vi "TelemGUI_v1_4.vi"(0 "Port number":refnum<visa-resource-name>="COM1", 1 "baud rate":u32=38400, 2 "data bits":u16=8 min=5 max=8 step=1, 3 "parity":u16(ring) items=["None", "Odd", "Even", "Mark", "Space"], 4 "stop bits":u16(ring)=10 items=["1.0"=10, "1.5"=15, "2.0"=20], 7 "flow control":u16(ring) items=["None"=0, "XON/XOFF"=1, "RTS/CTS"=2, "DTR/DSR"=4]) -> ()   [LabVIEW 2009]
doc: "McMaster Solar Car Project telemetry graphical front end for Spitfire (2014). Developed for telemetry circuit running firmware revision 6.\n\nINSTRUCTIONS:\n1. In the 'Configuration' tab, select the COM port which the radio is connected to (i.e. - the COM port which enumerated when the UART/receiver module was connected to the PC). If you connected the receiver after opening the GUI, select 'Refresh' from the drop down menu to refresh the COM port list.\n\n2. Set port options. For the current version of the Telemetry hardware using the XCite RF modules use 38400 baud, 8 data bits, parity none, 1 stop bit, flow control none\n\n3. Click on the folder icon next to the log file path dialog box. Select a save location and name for the log file. If you would like to add comments to the log file header, enter these in the 'Notes' dialog box. \n\n4. Select which battery pack is installed in the solar car in the \"Configuration\" tab by clicking the correct radio button (\"Race pack\" or \"Practice pack\"). This selection applies the correct conversion/calibration factors for the current sensor measurement on the battery pack. \n\n5. Click the 'Connect' button. If communication with the telemetry broadcast is successful, the \"heartbeat\" indicator in the window should flash once per full data receipt cycle (approximately once per second). As new data is received from the solar car, the indicators in the various tabs of the front panel will update.\n\n6. To disconnect from the radio link save the data log to file, press the 'Disconnect' button located below the GUI window.\n\n7. If the incorrect COM port was selected, you must first 'Disconnect' before changing the port settings. This also applies if you would like to change the name of the log file. Note that a delay of up to 2 seconds may occur when the 'Disconnect' button is pressed. Once disconnected, change the COM port options and/or the log file path and comment before clicking 'Connect' again.\n\n8. To end execution of the program, first click 'Disconnect' and then click 'Cancel.'\n\nUSAGE NOTES:\n- If the solar car is out of radio range, the telemetry front end displays the most recently received data. The front end will continue to update once the solar car transmitter re-enters radio range.\n\n- In the 'Overview' panel, the displayed 'Battery Charge' is either the charge or discharge capacity, depending on if the battery is charging or discharging. The charge capacity is the estimated state-of-charge of the most charged module in the battery pack; the discharge capacity is the state-of-charge of the least charged module in the battery pack. Both of these values are visible in the 'Battery Details' tab. \n\n- In practice, these two charge values will be different due to battery pack misbalance. A large difference between these two values is undesirable since the battery pack can only be discharged until the discharge capacity reaches 0 and can only be charged until the charge capacity reaches 1.\n\n- Also note that the battery charge is merely an estimate based on a simple battery model. The model predictions are poor above 95% and below 5% state of charge\n\n- The value for \"Range (km)\" is an estimate of the distance that can be travelled at the current rate of power draw from the battery pack before a battery protection system (BPS) trip will occur. The accuracy of this data is untested. This calculation uses the discharge capacity if the battery pack is being discharged, and vice-versa.\n\n- Negative values for range are reported if the battery pack is being charged while the car is driving (i.e. - during regen braking or if the solar array is producing more power than required by the motor).\n\n- Currently \"Economy (Wh/km)\" and \"Range (km)\" are calculated from instantaneous values based on most recently received data. Corrupted radio data will yield nonsensical results (i.e. - at the moment the solar car is leaving or re-entering radio range)."
uses:
  <vilib>/Instr/_visa.llb/VISA Configure Serial Port (Instr).vi
  <vilib>/express/express arith-compare/Formula/XNode/ExpressFormulaBlockNode.xnode
  <vilib>/express/express shared/transition.llb/Waveform Array To Dynamic.vi
  <vilib>/express/express shared/transition.llb/Dynamic To Waveform Array.vi
  <vilib>/express/express shared/ex_Modify Signal Name.vi
  <vilib>/express/express arith-compare/Formula/Block/exnFormulaBlock how many pts in the wave.vi
panel:
  out "Radio heartbeat":bool
  in  "?":T1(tab)
  out "Status message:":string="LabVIEW application is not running! Press Ctrl+R!"
  in  "Cancel Button":bool
  in  "CONNECT":bool
  in  "Battery pack calibration":enum32{"ALPHA", "ZAPPA"}(radio)
  in  "Full path to log file":path
  in  "Notes (appended to log file)":string
  in  "Disconnect":bool
  out "Cruising speed":dbl(slide) scale=0.0..120.0 scale format="%#.0f"
  out "Reverse":bool
  out "MPPT\nTemperature":dbl(slide) scale=0.0..60.0
  out "Net Power Usage (W)":dbl(slide) scale=-1000.0..1000.0
  out "Throttle position":dbl(slide) scale=0.0..1.0 scale format="%#.1f"
  out "Range (km)":dbl format="%.1f"
  out "Battery Charge":dbl(slide) scale=0.0..1.0
  out "Controller \nTemperature":dbl(slide) scale=0.0..60.0
  out "Battery\nTemperature":dbl(slide) scale=0.0..60.0
  out "Aux Error":bool
  out "Aux Low":bool
  out "Aux OK":bool
  out "Pack Hi":bool
  out "Pack Low":bool
  out "Pack OK":bool
  out "Array Amps":dbl format="%.1f"
  out "Motor Amps":dbl format="%.1g"
  out "Motor Power (W)":dbl(slide) scale=0.0..2000.0
  out "Array Power (W)":dbl(slide) scale=0.0..1200.0
  out "Bus Voltage (V)":dbl format="%.1f"
  out "Economy (Wh/km)":dbl format="%.1f"
  out "Speed (km/h)":dbl(knob) scale=0.0..100.0
  out "High temp":bool
  out "Over voltage":bool
  out "Under voltage":bool
  out "Min ID":i8 format="%02x"
  out "Max ID":i8 format="%02x"
  out "Min voltage":dbl format="%.2f"
  out "Max voltage":dbl format="%.2f"
  out "NET battery power (W)":dbl format="%.1f"
  out "MAIN Bus (A)":dbl format="%.1f"
  out "MAIN Bus (V)":dbl format="%.1f"
  out "Error":bool
  out "Low":bool
  out "OK":bool
  out "Max temp (ºC)":dbl(slide) scale=0.0..60.0
  out "AUX Bus (V)":dbl format="%.2f"
  out "Cell Voltages (V)":dbl[](array[numeric]) format="%.2f"
  out "Charge\nCapacity":dbl(slide) scale=0.0..1.0
  out "Discharge\nCapacity":dbl(slide) scale=0.0..1.0
  out "Voltage":dbl[](array[numeric]) format="%.2f"
  out "Temp":dbl[](array[numeric])
  out "BPS total voltage":dbl
  out "MPPT Temp (ºC)":dbl
  out "Power (W)":dbl format="%0.1f"
  out "Current (A)":dbl format="%0.1f"
  out "Voltage (V)":dbl format="%0.1f"
  out "MPPT Temp (ºC)":dbl
  out "Power (W)":dbl format="%0.1f"
  out "Current (A)":dbl format="%0.1f"
  out "Voltage (V)":dbl format="%0.1f"
  out "MPPT Temp (ºC)":dbl
  out "Power (W)":dbl format="%0.1f"
  out "Current (A)":dbl format="%0.1f"
  out "Voltage (V)":dbl format="%0.1f"
  out "MPPT Temp (ºC)":dbl
  out "Power (W)":dbl format="%0.1f"
  out "Current (A)":dbl format="%0.1f"
  out "Voltage (V)":dbl format="%0.1f"
  out "NET OUTPUT (W)":dbl format="%6.1f"
  out "Output current (A)":dbl format="%.1f"
  out "Output voltage (V)":dbl format="%.1f"
  out "Drive Velocity":dbl
  out "Drive Current":dbl format="%.2f"
  out "DSP Temp":dbl
  out "HS Temp":dbl
  out "RPM":dbl
  out "Bus Curr":dbl format="%.1f"
  out "Bus Volt":dbl format="%.1f"
  out "ArrayCurr":dbl
  out "AuxCell":dbl[](array[numeric])
  out "Temp":dbl[](array[numeric])
  out "Volt Out":dbl[](array[numeric])
  out "Curr In":dbl[](array[numeric])
  out "Volt In":dbl[](array[numeric])
  out "Current":dbl
  out "Temp":dbl[](array[numeric])
  out "Radio receive buffer":string
  out "Volt":dbl[](array[numeric])
  out "Selected COM port":refnum<visa-resource-name>
  out "COM error out":errorcluster
  out "Logfile handle":refnum<file>
  # "2014 Telemetry GUI v1.4"
  # "For additional information select File >> VI Properties >> Documentation"
  # "NOTE - Default port settings are:\nBaud rate: 38400\nData bits: 8\nParity: none\nStop bits: 1\nFlow control: none"
  # "Voltage Status"
  # "Pack module readings"
  # "Pack status and warnings"
  # "0x00"
  # "0x01"
  # "0x02"
  # "0x03"
  # "0x04"
  # "0x05"
  # "0x06"
  # "0x07"
  # "0x08"
  # "0x09"
  # "0x0A"
  # "0x0B"
  # "0x0C"
  # "0x0D"
  # "0x0E"
  # "0x0F"
  # "0x10"
  # "0x11"
  # "Cell 0"
  # "0x12"
  # "Cell 1"
  # "0x13"
  # "Cell 2"
  # "0x14"
  # "0x15"
  # "Cell 3"
  # "0x16"
  # "0x17"
  # "0x18"
  # "0x19"
  # "BANK A"
  # "BANK B"
  # "BANK A"
  # "BANK B"
  # "BANK C"
  # "BANK D"
  # "BANK C"
  # "BANK D"
  # "Raw analog data"
  # "MPPT raw data"
  # "BPS raw data"
  # "0001"
  # "0010"
  # "0x00"
  # "0011"
  # "0x01"
  # "0100"
  # "0x02"
  # "0x03"
  # "0x04"
  # "Tritium/Drive raw data"
  # "0x05"
  # "0x06"
  # "0x07"
  # "0x08"
  # "0x09"
  # "0x0A"
  # "0x0B"
  # "0x0C"
  # "0x0D"
  # "0x0E"
  # "0x0F"
  # "0x10"
  # "0x11"
  # "0x12"
  # "0x13"
  # "0x14"
  # "0x15"
  # "0x16"
  # "0x17"
  # "0x18"
  # "0x19"
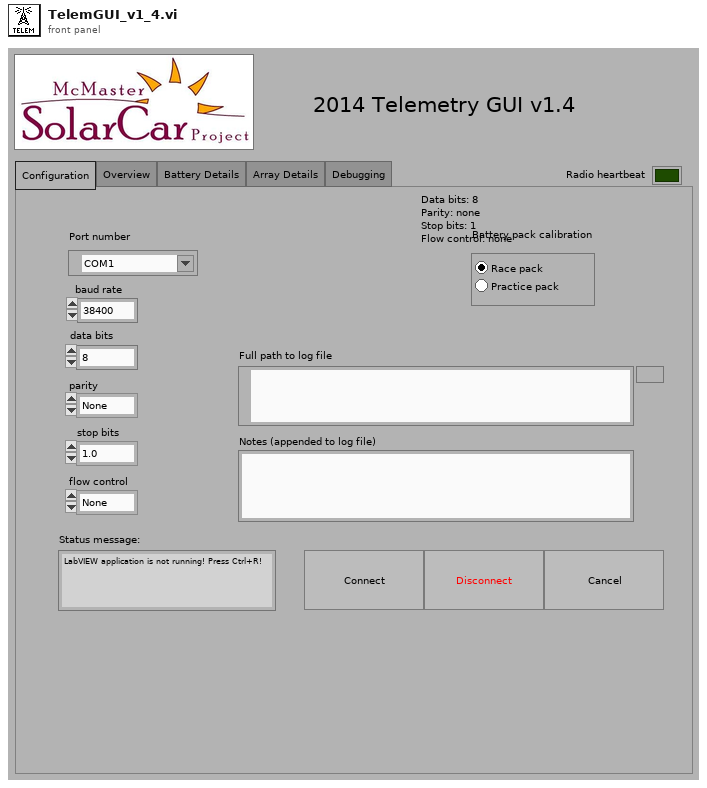
[diagram p1: front panel]
types:
  T1 = enum32{"Configuration", "Overview", "Battery Details", "Array Details", "Debugging"}
  T2 = enum16{"open", "replace", "create", "open or create", "replace or create", "replace or create with confirmation"}
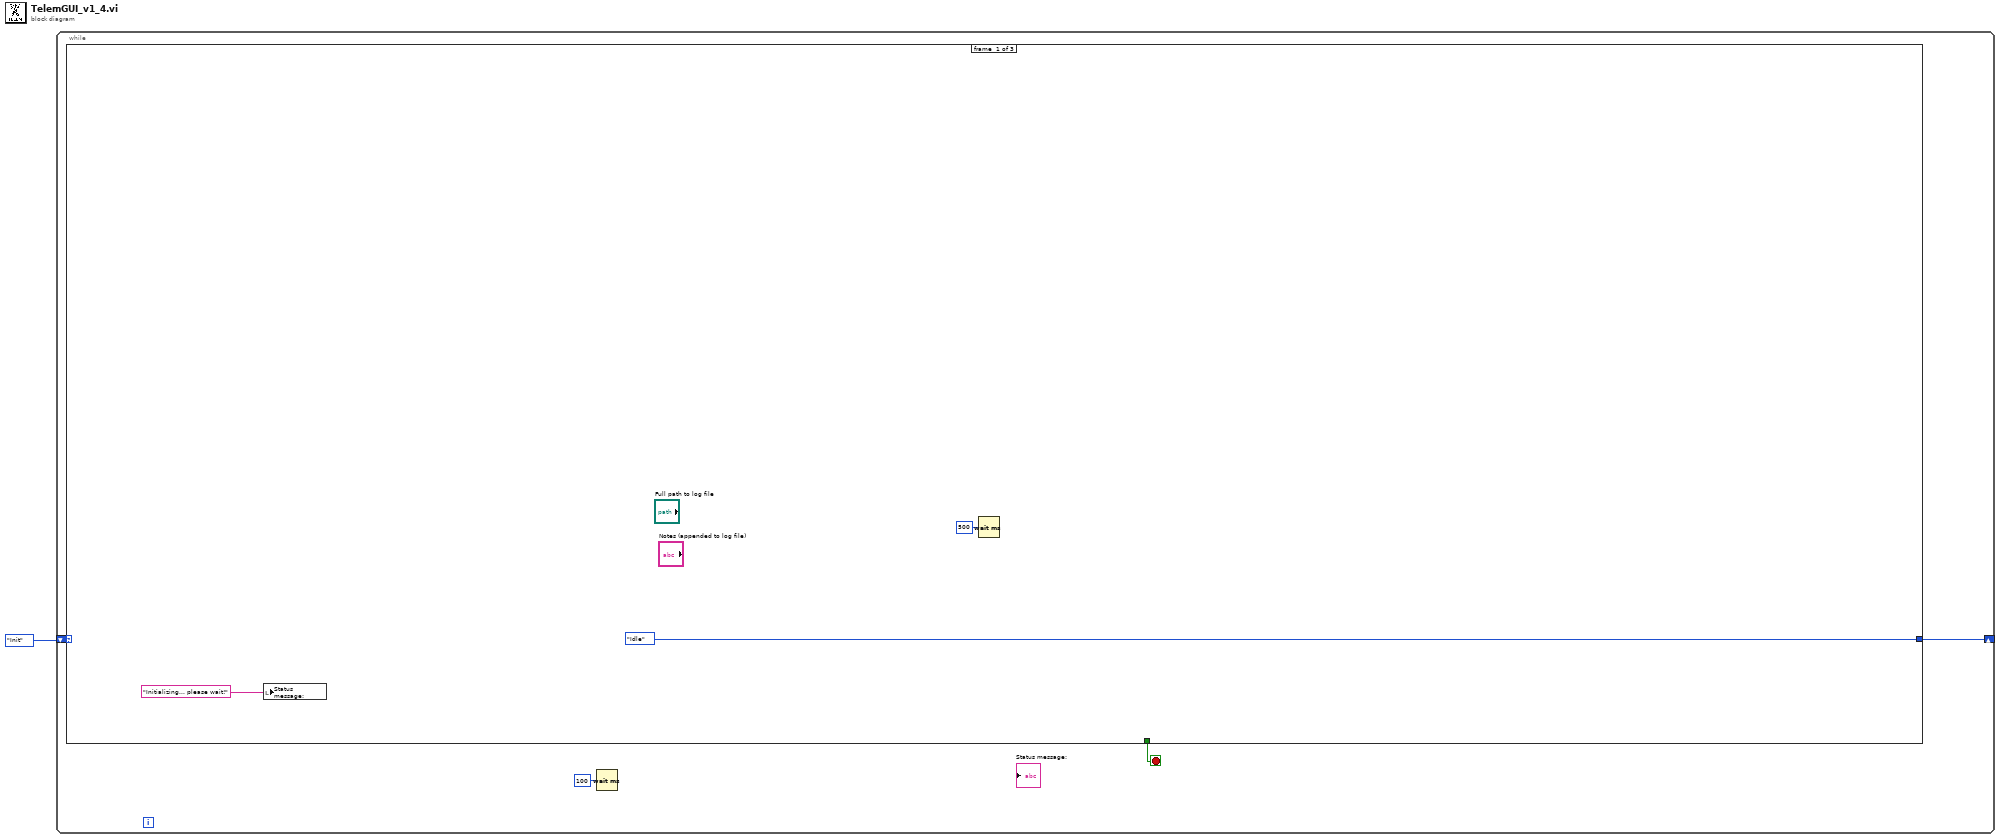
[diagram p0: block diagram]
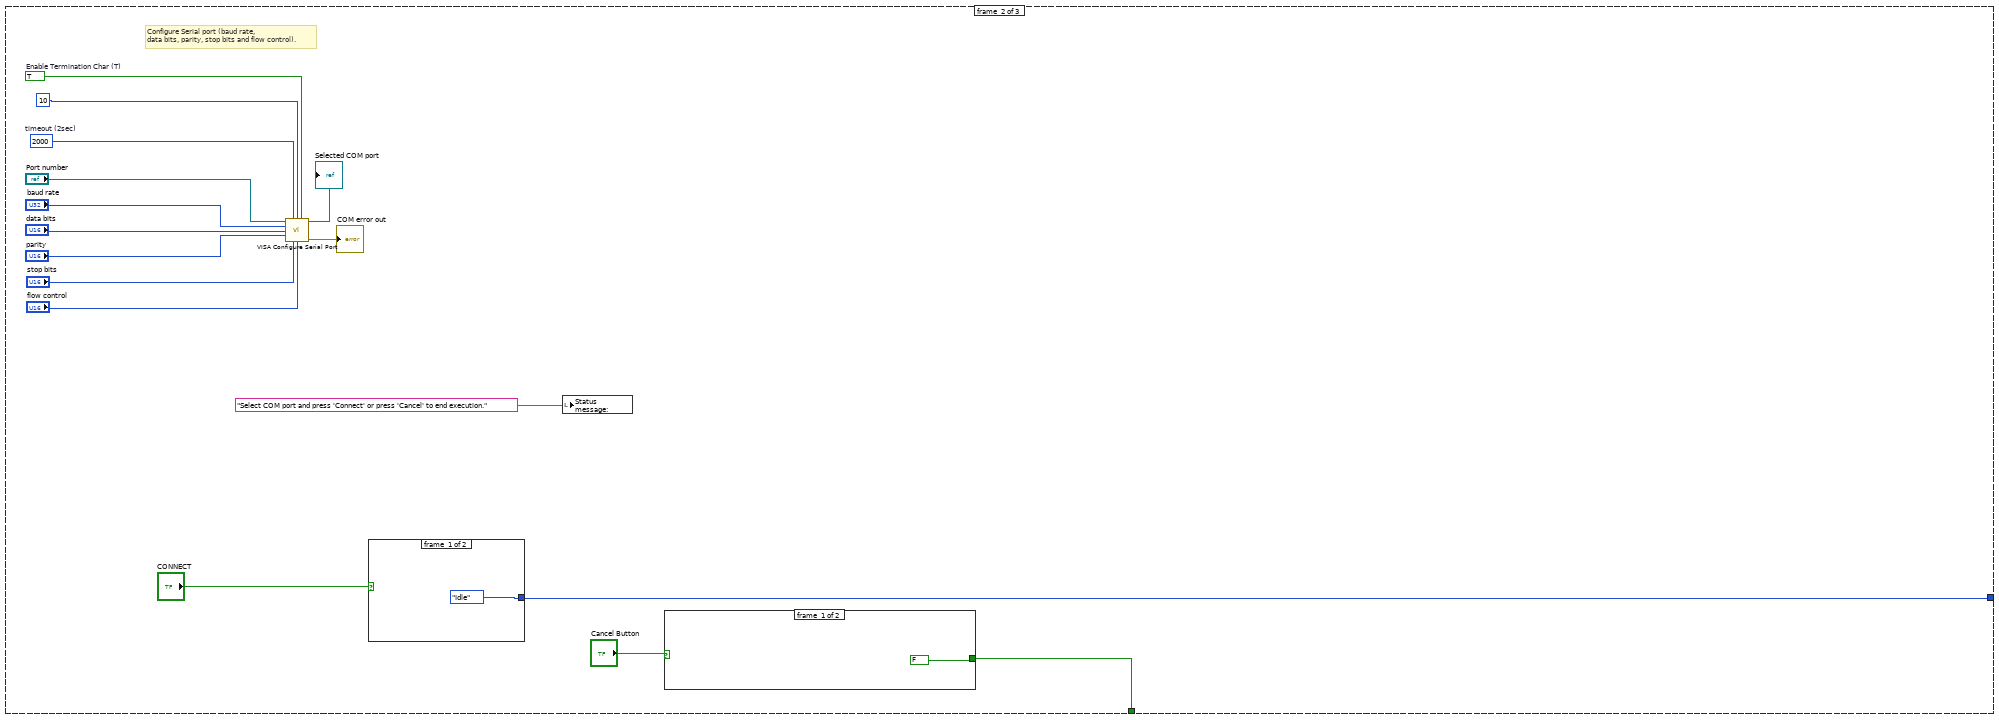
[diagram p2: hidden frame]
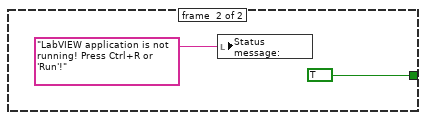
[diagram p3: hidden frame]
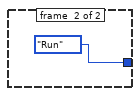
[diagram p4: hidden frame]
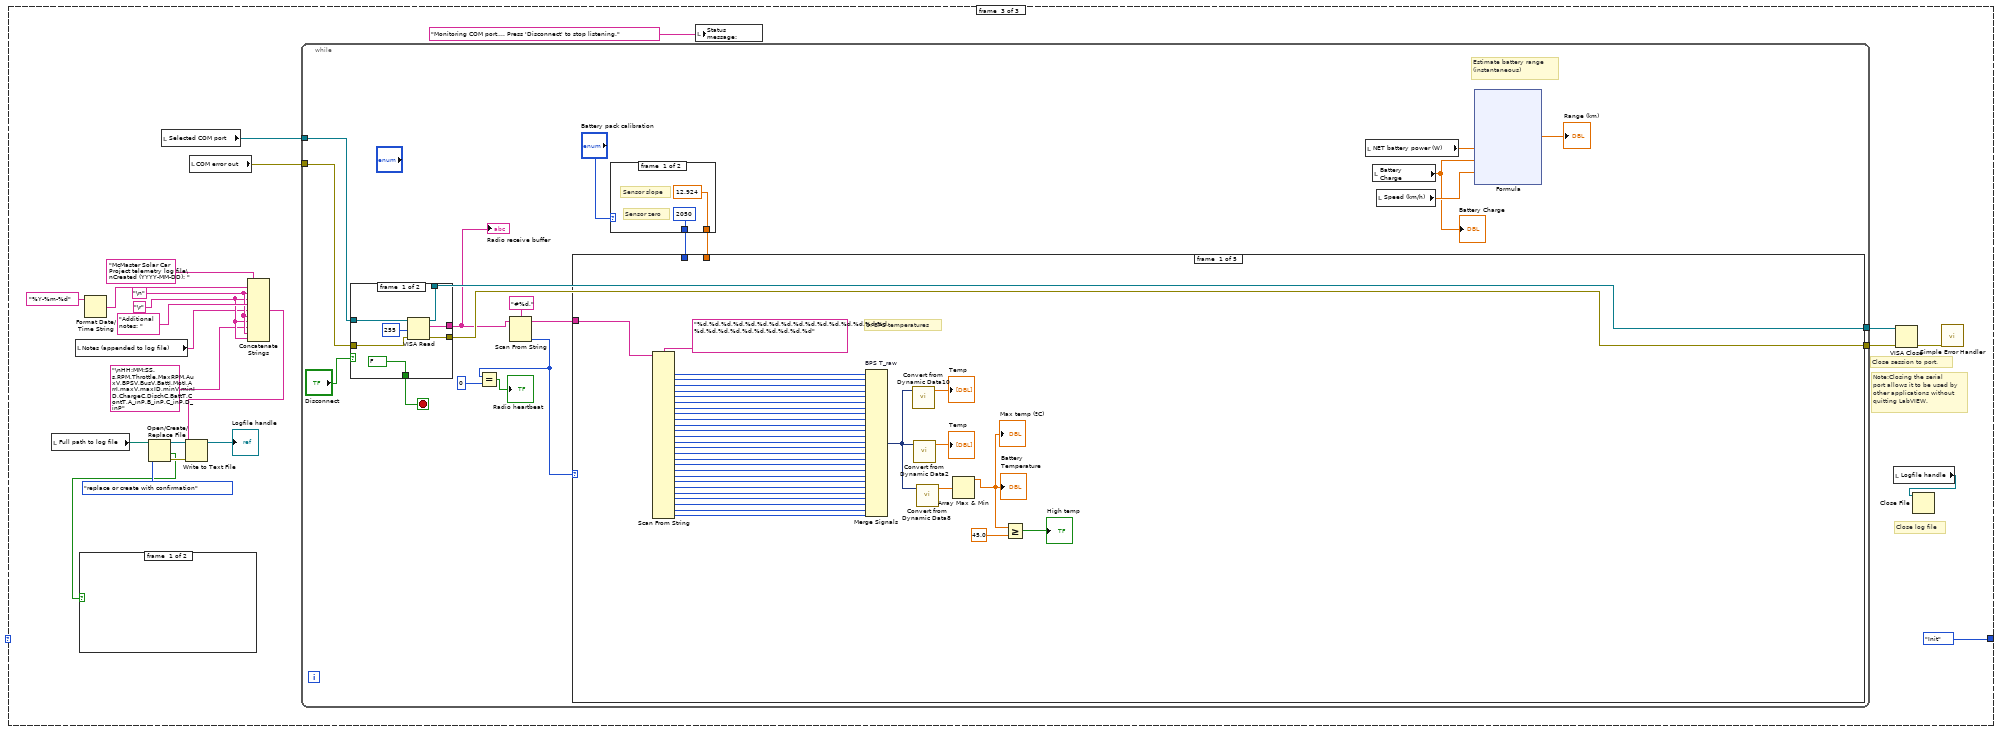
[diagram p5: hidden frame]
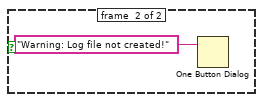
[diagram p6: hidden frame]
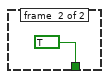
[diagram p7: hidden frame]
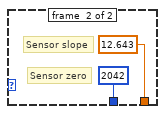
[diagram p8: hidden frame]
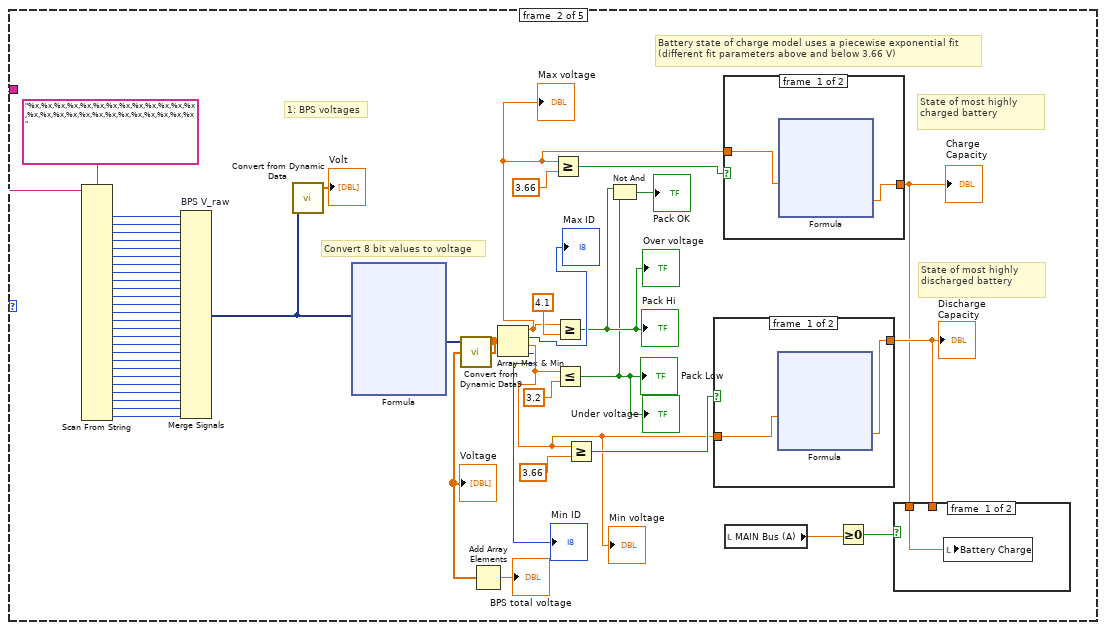
[diagram p9: hidden frame]
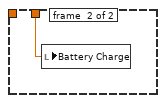
[diagram p10: hidden frame]
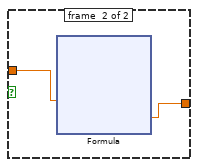
[diagram p11: hidden frame]
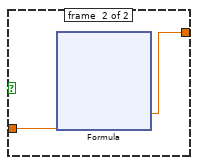
[diagram p12: hidden frame]
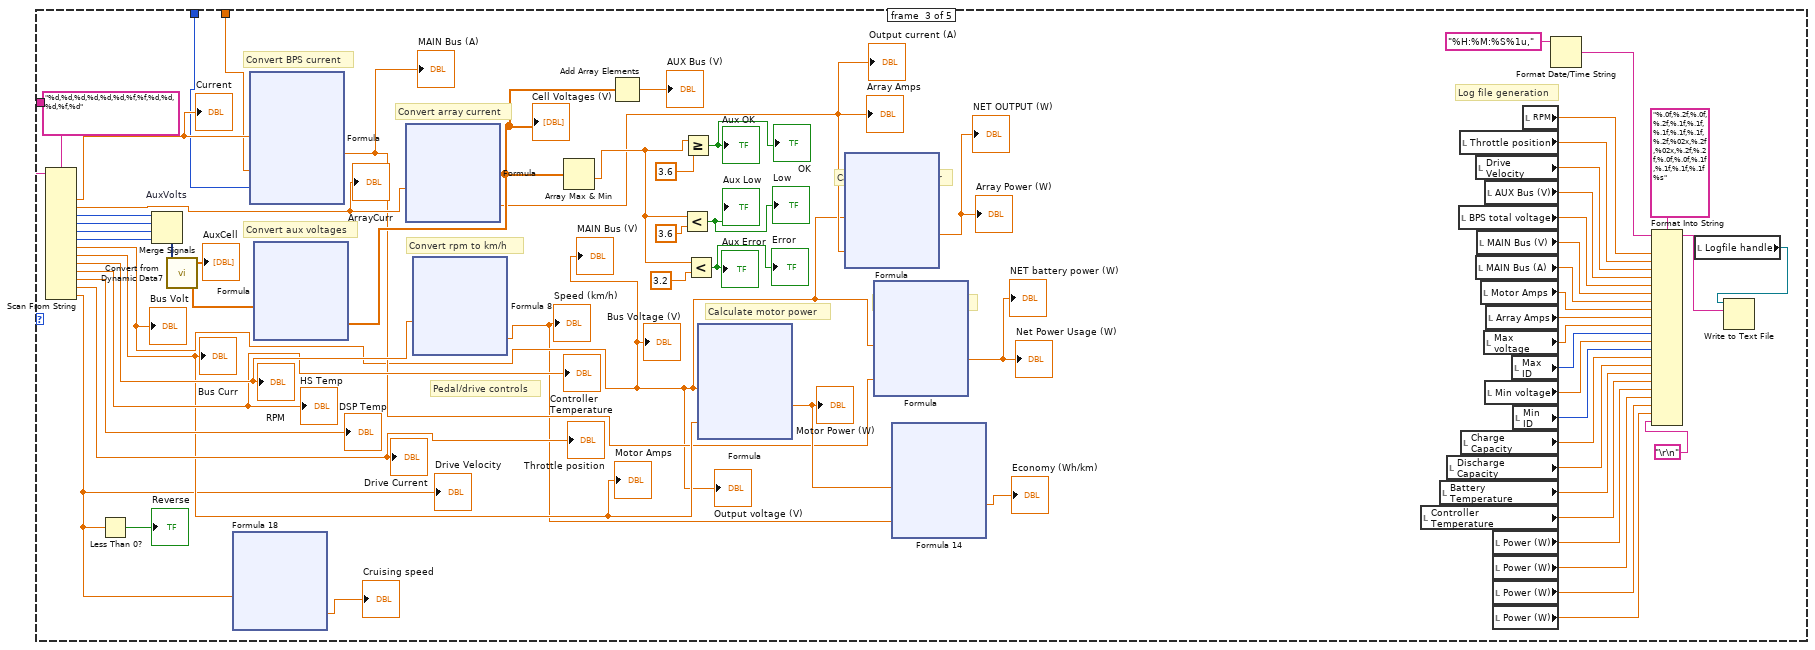
[diagram p13: hidden frame]
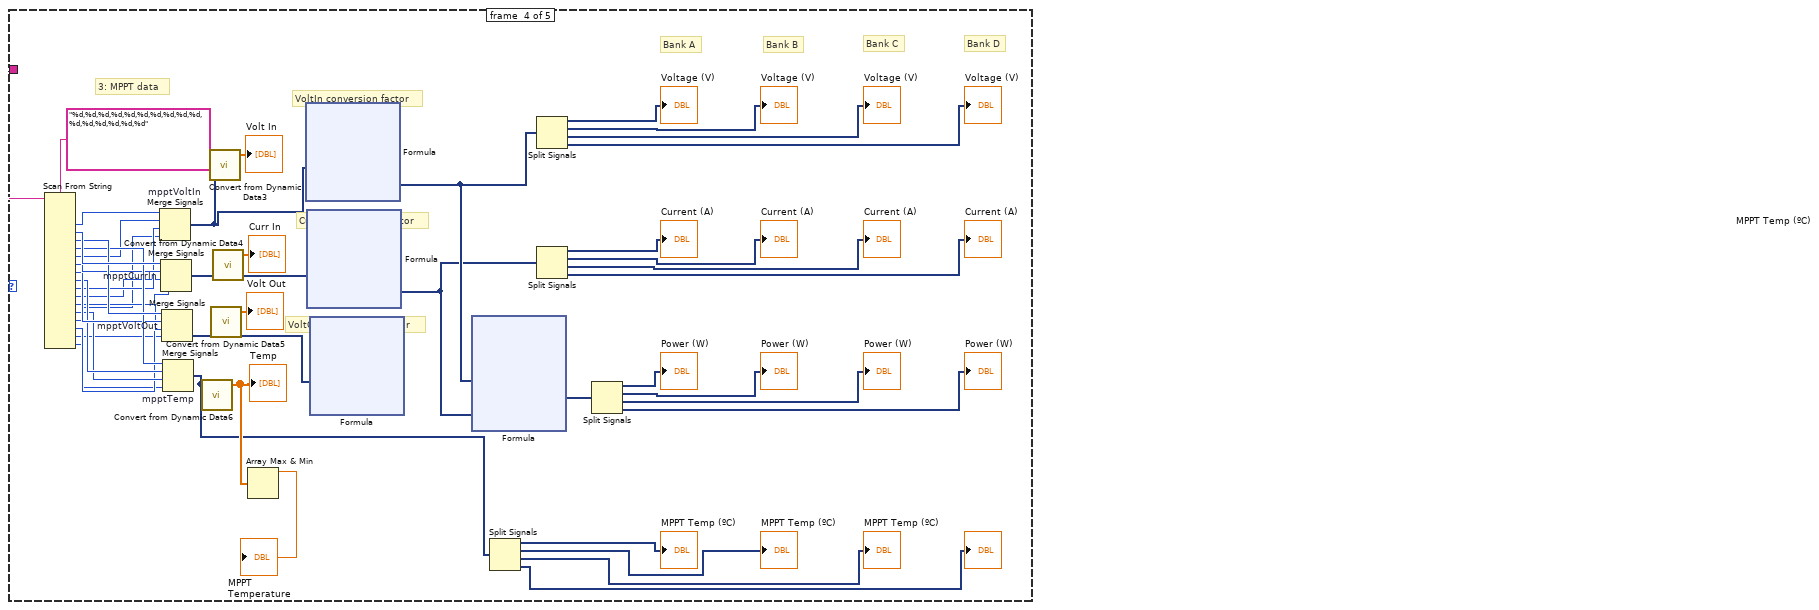
[diagram p14: hidden frame]
diagram:
  n1 = while {
    shift-right: [w4] -> _
    shift-left: enum16{"Init", "Idle", "Run"}."Init" -> [w5]
    stop <- w2 stop-if-true
    n2 = case shown="\"Run\"" w5 {
      tunnel: [enum16{"Init", "Idle", "Run"}."Idle" w23 enum16{"Init", "Idle", "Run"}."Init"] -> w4
      tunnel: [_ w20 _] -> w2
      frame #0 {
        n3 = local write "Status message:"("Initializing... please wait!" ("Status message:")) -> ()
        n4 = Wait (ms)(milliseconds to wait=u32 500) -> ()  [unwired: 1 out]
      }
      frame #1 {
        w15 = TRUE  # Enable Termination Char (T)
        w14 = u32 2000  # timeout (2sec)
        # "Configure Serial port (baud rate,\ndata bits, parity, stop bits and flow control)."
        n5 = call-poly "VISA Configure Serial Port"("VISA resource name"="Port number", "timeout (10sec)"=w14, "termination char\n(0xA = '\\n' = LF)"=10, "Enable Termination\nChar (T)"=w15, "baud rate (9600)"="baud rate", "data bits (8)"="data bits", "parity (0:none)"="parity", "stop bits (10: 1 bit)"="stop bits", "flow control (0:none)"="flow control") -> ("VISA resource name out"=→"Selected COM port":refnum<visa-resource-name>, "error out"=→"COM error out":errorcluster)  [unwired: 5 in]
        n6 = case shown="False" "CONNECT" {
          tunnel: [enum16{"Init", "Idle", "Run"}."Idle" enum16{"Init", "Idle", "Run"}."Run"] -> w23
          frame #0 {
          }
          frame #1 {
          }
        }
        n7 = local write "Status message:"("Select COM port and press 'Connect' or press 'Cancel' to end execution." ("Status")) -> ()
        n8 = case shown="True" "Cancel Button" {
          tunnel: [FALSE TRUE] -> w20
          frame #0 {
          }
          frame #1 {
            n9 = local write "Status message:"("LabVIEW application is not running! Press Ctrl+R or 'Run'!" ("Status")) -> ()
          }
        }
      }
      frame #2 {
        w39 = "\n"
        w38 = "\r"
        # "Close log file"
        # "Note:Closing the serial port allows it to be used by other applications without\nquitting LabVIEW."
        # "Close session to port."
        n10 = local read "Full path to log file"() -> (w45:path)
        n11 = local read "Notes (appended to log file)"() -> (w34:string)
        n12 = Format Date/Time String(time format string (%c)="%Y-%m-%d") -> (date/time string=w41:string)  [unwired: 2 in]
        n13 = Open/Create/Replace File(file path (use dialog)=w45, operation (0:open)=T2."replace or create with confirmation") -> (refnum out=w48:refnum<file>, cancelled=w44:bool, error out=w47:errorcluster)  [unwired: 4 in]
        n14 = case shown="True" w44 {
          frame #0 {
          }
          frame #1 {
            n15 = One Button Dialog ("Log creation cancelled")(message="Warning: Log file not created!") -> ()  [unwired: 1 in, 1 out]
          }
        }
        n16 = local read "Selected COM port"() -> (w37:refnum<visa-resource-name>)
        n17 = local read "COM error out"() -> (w36:errorcluster)
        n18 = Concatenate Strings("McMaster Solar Car Project telemetry log file\nCreated (YYYY-MM-DD): ", w41, w39, w38, "Additional notes: " ("string"), w34, w39, w38, "\nHH:MM:SS.s,RPM,Throttle,MaxRPM,AuxV,BPSV,BusV,BattI,MotI,ArrI,maxV,maxID,minV,minID,ChargeC,DischC,BattT,ContT,A_inP,B_inP,C_inP,D_inP" ("string"), w39, w38) -> (w35:string)
        n19 = Write to Text File(file (use dialog)=w48, text=w35, error in=w47) -> (refnum out=→"Logfile handle":refnum<file>)  [unwired: 1 in, 2 out]
        n20 = while {
          tunnel: [w58] -> w50
          tunnel: [w59] -> w51
          tunnel: w37 -> [w55]
          tunnel: w36 -> [w54]
          stop <- w56 stop-if-true
          # "Estimate battery range\n(instantaneous)"
          n21 = case shown="False" "Disconnect" {
            tunnel: w55 -> [w78 _]
            tunnel: w54 -> [w77 _]
            tunnel: [w76 _] -> w59
            tunnel: [w75 _] -> w58
            tunnel: [w74 _] -> w57
            tunnel: [FALSE TRUE] -> w56
            frame #0 {
              n22 = VISA Read(VISA resource name=w78, byte count=255, error in (no error)=w77) -> (VISA resource name out=w76:refnum<visa-resource-name>, read buffer=w74:string, error out=w75:errorcluster)  [unwired: 1 out]
            }
            frame #1 {
            }
          }
          "Radio receive buffer" <- w57
          n23 = Scan From String(format string="#%d,", input string=w57) -> (remaining string=w71:string, output 1=w70:i32)  [unwired: 3 in, 2 out]
          n24 = Equal?(x=w70, y=0) -> (x = y?=→"Radio heartbeat":bool)
          n25 = case shown="\"ALPHA\", Default" "Battery pack calibration" {
            tunnel: [12.924 12.643] -> w66
            tunnel: [2050 2042] -> w65
            frame #0 {
              # "Sensor zero"
              # "Sensor slope"
            }
            frame #1 {
              # "Sensor zero"
              # "Sensor slope"
            }
          }
          n26 = case shown="2" w70 {
            tunnel: w71 -> [w131 w180 w425 w557 _]
            tunnel: w66 -> [_ _ w400 _ _]
            tunnel: w65 -> [_ _ w399 _ _]
            frame #0 {
              # "0: BPS temperatures"
              n27 = Scan From String(format string="%d,%d,%d,%d,%d,%d,%d,%d,%d,%d,%d,%d,%d,%d,%d,%d,%d,%d,%d,%d,%d,%d,%d,%d,%d,%d", input string=w131) -> (output 1=w129:i32, output 2=w128:i32, output 3=w127:i32, output 4=w126:i32, output 5=w125:i32, output 6=w124:i32, output 7=w123:i32, output 8=w122:i32, output 9=w121:i32, output 10=w120:i32, output 11=w119:i32, output 12=w118:i32, output 13=w117:i32, output 14=w116:i32, output 15=w115:i32, output 16=w114:i32, output 17=w113:i32, output 18=w112:i32, output 19=w111:i32, output 20=w110:i32, output 21=w109:i32, output 22=w108:i32, output 23=w107:i32, output 24=w104:i32, output 25=w106:i32, output 26=w105:i32)  [unwired: 28 in, 3 out]
              n28 = Merge Signals "BPS T_raw"(w129, w128, w127, w126, w125, w124, w123, w122, w121, w120, w119, w118, w117, w116, w115, w114, w113, w112, w111, w110, w109, w108, w107, w104, w106, w105) -> (w102:dynamicdata)
              n29 = call "Convert from Dynamic Data10"("Dynamic Data Type"=w102) -> ("Array"=→"Temp":dbl[])  [unwired: 3 in]
              n30 = call "Convert from Dynamic Data2"("Dynamic Data Type"=w102) -> ("Array"=→"Temp":dbl[])  [unwired: 3 in]
              n31 = call "Convert from Dynamic Data8"("Dynamic Data Type"=w102) -> ("Array"=w97:dbl[])  [unwired: 3 in]
              n32 = Array Max & Min(array=w97) -> (max value=w100:dbl)  [unwired: 3 out]
              "Battery\nTemperature" <- w100
              "Max temp (ºC)" <- w100
              n33 = Greater Or Equal?(x=w100, y=45.0) -> (x >= y?=→"High temp":bool)
            }
            frame #1 {
              # "State of most highly discharged battery"
              # "State of most highly charged battery"
              # "Battery state of charge model uses a piecewise exponential fit\n(different fit parameters above and below 3.66 V)"
              # "1: BPS voltages"
              # "Convert 8 bit values to voltage"
              n34 = Scan From String(format string="%x,%x,%x,%x,%x,%x,%x,%x,%x,%x,%x,%x,%x,%x,%x,%x,%x,%x,%x,%x,%x,%x,%x,%x,%x,%x", input string=w180) -> (output 1=w179:i32, output 2=w178:i32, output 3=w177:i32, output 4=w176:i32, output 5=w175:i32, output 6=w174:i32, output 7=w173:i32, output 8=w172:i32, output 9=w171:i32, output 10=w170:i32, output 11=w169:i32, output 12=w168:i32, output 13=w167:i32, output 14=w166:i32, output 15=w165:i32, output 16=w164:i32, output 17=w163:i32, output 18=w162:i32, output 19=w161:i32, output 20=w160:i32, output 21=w159:i32, output 22=w154:i32, output 23=w158:i32, output 24=w157:i32, output 25=w156:i32, output 26=w155:i32)  [unwired: 28 in, 3 out]
              n35 = Merge Signals "BPS V_raw"(w179, w178, w177, w176, w175, w174, w173, w172, w171, w170, w169, w168, w167, w166, w165, w164, w163, w162, w161, w160, w159, w154, w158, w157, w156, w155) -> (w153:dynamicdata)
              n36 = call "Convert from Dynamic Data"("Dynamic Data Type"=w153) -> ("Array"=→"Volt":dbl[])  [unwired: 3 in]
              n37 = xnode "Formula"("X1"=w153) -> ("Result"=w151:dynamicdata)  [unwired: 1 in, 1 out]
              n38 = call "Convert from Dynamic Data9"("Dynamic Data Type"=w151) -> ("Array"=w133:dbl[])  [unwired: 3 in]
              "Voltage" <- w133
              n39 = Add Array Elements(numeric array=w133) -> (sum=→"BPS total voltage":dbl)
              n40 = Array Max & Min(array=w133) -> (max value=w143:dbl, max index (indices)=→"Max ID":i32, min value=w142:dbl, min index (indices)=→"Min ID":i32)
              "Max voltage" <- w143
              "Min voltage" <- w142
              n41 = Greater Or Equal?(x=w143, y=3.66) -> (x >= y?=w144:bool)
              n42 = Greater Or Equal?(x=w143, y=4.1) -> (x >= y?=w139:bool)
              "Pack Hi" <- w139
              "Over voltage" <- w139
              n43 = Less Or Equal?(x=w142, y=3.2) -> (x <= y?=w138:bool)
              "Pack Low" <- w138
              "Under voltage" <- w138
              n44 = Greater Or Equal?(x=w142, y=3.66) -> (x >= y?=w146:bool)
              n45 = Not And(1:w138, 2:w139) -> (0:→"Pack OK":bool)
              n46 = case shown="False" w146 {
                tunnel: w142 -> [w205 w215]
                tunnel: [w204 w214] -> w135
                frame #0 {
                  n47 = xnode "Formula"("X1"=w205) -> ("Result"=w204:dbl)  [unwired: 1 in, 1 out]
                }
                frame #1 {
                  n48 = xnode "Formula"("X1"=w215) -> ("Result"=w214:dbl)  [unwired: 1 in, 1 out]
                }
              }
              "Discharge\nCapacity" <- w135
              n49 = case shown="False" w144 {
                tunnel: [w185 w195] -> w134
                tunnel: w143 -> [w184 w194]
                frame #0 {
                  n50 = xnode "Formula"("X1"=w184) -> ("Result"=w185:dbl)  [unwired: 1 in, 1 out]
                }
                frame #1 {
                  n51 = xnode "Formula"("X1"=w194) -> ("Result"=w195:dbl)  [unwired: 1 in, 1 out]
                }
              }
              "Charge\nCapacity" <- w134
              n52 = local read "MAIN Bus (A)"() -> (w137:dbl)
              n53 = Greater Or Equal To 0?(x=w137) -> (x >= 0?=w136:bool)
              n54 = case shown="True" w136 {
                tunnel: w135 -> [_ w183]
                tunnel: w134 -> [w182 _]
                frame #0 {
                  n55 = local write "Battery Charge"(w182) -> ()
                }
                frame #1 {
                  n56 = local write "Battery Charge"(w183) -> ()
                }
              }
            }
            frame #2 {
              # "Log file generation"
              # "Calculate array power"
              # "Battery (net) power"
              # "Calculate motor power"
              # "Convert rpm to km/h"
              # "Pedal/drive controls"
              # "Convert aux voltages"
              # "Convert array current"
              # "Convert BPS current"
              n57 = Scan From String(format string="%d,%d,%d,%d,%d,%d,%f,%f,%d,%d,%d,%f,%d", input string=w425) -> (output 1=w420:dbl, output 2=w417:dbl, output 3=w424:i32, output 4=w423:i32, output 5=w422:i32, output 6=w421:i32, output 7=w392:dbl, output 8=w410:dbl, output 9=w415:dbl, output 10=→"HS Temp" →"Controller \nTemperature":dbl, output 11=→"DSP Temp":dbl, output 12=→"Drive Current" →"Throttle position":dbl, output 13=w402:dbl)  [unwired: 15 in, 3 out]
              "Current" <- w420
              "ArrayCurr" <- w417
              "Bus Volt" <- w392
              "Bus Curr" <- w410
              "RPM" <- w415
              "Drive Velocity" <- w402
              "Motor Amps" <- w410
              "Bus Voltage (V)" <- w392
              "Output voltage (V)" <- w392
              "MAIN Bus (V)" <- w392
              n58 = Less Than 0?(x=w402) -> (x < 0?=→"Reverse":bool)
              n59 = Merge Signals "AuxVolts"(w424, w423, w422, w421) -> (w419:dynamicdata)
              n60 = call "Convert from Dynamic Data7"("Dynamic Data Type"=w419) -> ("Array"=w418:dbl[])  [unwired: 3 in]
              "AuxCell" <- w418
              n61 = xnode "Formula 18"("RPM"=w402) -> ("Result"=→"Cruising speed":dbl)  [unwired: 1 in, 1 out]
              n62 = xnode "Formula"("battADC"=w420, "hallSlope"=w400, "hallZero"=w399) -> ("Result"=w393:dbl)  [unwired: 1 in, 1 out]
              "MAIN Bus (A)" <- w393
              n63 = xnode "Formula"("X1"=w418) -> ("Result"=w406:dbl[])  [unwired: 1 in, 1 out]
              "Cell Voltages (V)" <- w406
              n64 = xnode "Formula"("ArrayADC"=w417) -> ("Result"=w397:dbl)  [unwired: 1 in, 1 out]
              "Array Amps" <- w397
              "Output current (A)" <- w397
              n65 = xnode "Formula 8"("RPM"=w415) -> ("Result"=w390:dbl)  [unwired: 1 in, 1 out]
              "Speed (km/h)" <- w390
              n66 = Array Max & Min(array=w406) -> (min value=w404:dbl)  [unwired: 3 out]
              n67 = Add Array Elements(numeric array=w406) -> (sum=→"AUX Bus (V)":dbl)
              n68 = Less?(x=w404, y=3.6) -> (x < y?=→"Aux Low" →"Low":bool)
              n69 = Greater Or Equal?(x=w404, y=3.6) -> (x >= y?=→"Aux OK" →"OK":bool)
              n70 = Less?(x=w404, y=3.2) -> (x < y?=→"Aux Error" →"Error":bool)
              n71 = xnode "Formula"("BusVolt"=w392, "MotCurr"=w410) -> ("Result"=w409:dbl)  [unwired: 1 in, 1 out]
              "Motor Power (W)" <- w409
              n72 = xnode "Formula"("BusVolt"=w392, "ArrayCurr"=w397) -> ("Result"=→"Array Power (W)" →"NET OUTPUT (W)":dbl)  [unwired: 1 in, 1 out]
              n73 = xnode "Formula"("busVolt"=w392, "battCurr"=w393) -> ("Result"=→"Net Power Usage (W)" →"NET battery power (W)":dbl)  [unwired: 1 in, 1 out]
              n74 = xnode "Formula 14"("MotW"=w409, "Speed"=w390) -> ("Result"=→"Economy (Wh/km)":dbl)  [unwired: 1 in, 1 out]
              n75 = local read "Controller \nTemperature"() -> (w368:dbl)
              n76 = local read "Battery\nTemperature"() -> (w369:dbl)
              n77 = local read "Discharge\nCapacity"() -> (w370:dbl)
              n78 = local read "BPS total voltage"() -> (w382:dbl)
              n79 = local read "Throttle position"() -> (w385:dbl)
              n80 = local read "Charge\nCapacity"() -> (w371:dbl)
              n81 = local read "Drive Velocity"() -> (w384:dbl)
              n82 = local read "MAIN Bus (A)"() -> (w380:dbl)
              n83 = local read "MAIN Bus (V)"() -> (w381:dbl)
              n84 = local read "Motor Amps"() -> (w378:dbl)
              n85 = local read "Max voltage"() -> (w379:dbl)
              n86 = local read "AUX Bus (V)"() -> (w383:dbl)
              n87 = local read "Min voltage"() -> (w373:dbl)
              n88 = local read "Array Amps"() -> (w377:dbl)
              n89 = local read "Power (W)"() -> (w367:dbl)
              n90 = local read "Power (W)"() -> (w366:dbl)
              n91 = local read "Power (W)"() -> (w365:dbl)
              n92 = local read "Power (W)"() -> (w364:dbl)
              n93 = local read "Max ID"() -> (w374:i8)
              n94 = local read "Min ID"() -> (w372:i8)
              n95 = local read "RPM"() -> (w386:dbl)
              n96 = Format Date/Time String(time format string (%c)="%H:%M:%S%1u,") -> (date/time string=w389:string)  [unwired: 2 in]
              n97 = Format Into String(format string="%.0f,%.2f,%.0f,%.2f,%.1f,%.1f,%.1f,%.1f,%.1f,%.2f,%02x,%.2f,%02x,%.2f,%.2f,%.0f,%.0f,%.1f,%.1f,%.1f,%.1f %s", initial string=w389, w386, w385, w384, w383, w382, w381, w380, w378, w377, w379, w374, w373, w372, w371, w370, w369, w368, w367, w366, w365, w364, "\r\n") -> (resulting string=w376:string)  [unwired: 1 in, 1 out]
              n98 = local read "Logfile handle"() -> (w375:refnum<file>)
              n99 = Write to Text File(file (use dialog)=w375, text=w376) -> ()  [unwired: 2 in, 3 out]
            }
            frame #3 {
              # "Power In"
              # "Bank D"
              # "Bank C"
              # "Bank B"
              # "Bank A"
              # "VoltOut conversion factor"
              # "CurrIn conversion factor"
              # "VoltIn conversion factor"
              # "3: MPPT data"
              n100 = Scan From String(format string="%d,%d,%d,%d,%d,%d,%d,%d,%d,%d,%d,%d,%d,%d,%d,%d", input string=w557) -> (output 1=w556:i32, output 2=w555:i32, output 3=w554:i32, output 4=w553:i32, output 5=w552:i32, output 6=w551:i32, output 7=w550:i32, output 8=w549:i32, output 9=w548:i32, output 10=w547:i32, output 11=w546:i32, output 12=w545:i32, output 13=w544:i32, output 14=w543:i32, output 15=w542:i32, output 16=w541:i32)  [unwired: 18 in, 3 out]
              n101 = Merge Signals "mpptVoltIn"(w556, w552, w548, w544) -> (w540:dynamicdata)
              n102 = Merge Signals "mpptCurrIn"(w555, w551, w547, w543) -> (w538:dynamicdata)
              n103 = Merge Signals "mpptVoltOut"(w554, w550, w546, w542) -> (w536:dynamicdata)
              n104 = Merge Signals "mpptTemp"(w553, w549, w545, w541) -> (w513:dynamicdata)
              n105 = call "Convert from Dynamic Data6"("Dynamic Data Type"=w513) -> ("Array"=w534:dbl[])  [unwired: 3 in]
              "Temp" <- w534
              n106 = call "Convert from Dynamic Data3"("Dynamic Data Type"=w540) -> ("Array"=→"Volt In":dbl[])  [unwired: 3 in]
              n107 = call "Convert from Dynamic Data5"("Dynamic Data Type"=w536) -> ("Array"=→"Volt Out":dbl[])  [unwired: 3 in]
              n108 = call "Convert from Dynamic Data4"("Dynamic Data Type"=w538) -> ("Array"=→"Curr In":dbl[])  [unwired: 3 in]
              n109 = Array Max & Min(array=w534) -> (max value=→"MPPT\nTemperature":dbl)  [unwired: 3 out]
              n110 = xnode "Formula"("X1"=w540) -> ("Result"=w532:dynamicdata)  [unwired: 1 in, 1 out]
              n111 = xnode "Formula"("X1"=w538) -> ("Result"=w530:dynamicdata)  [unwired: 1 in, 1 out]
              n112 = xnode "Formula"("X1"=w536) -> ()  [unwired: 1 in, 2 out]
              n113 = xnode "Formula"("VoltIn"=w532, "CurrIn"=w530) -> ("Result"=w531:dynamicdata)  [unwired: 1 in, 1 out]
              n114 = Split Signals(w513) -> (→"MPPT Temp (ºC)":dynamicdata, →"MPPT Temp (ºC)":dynamicdata, →"MPPT Temp (ºC)":dynamicdata, →"MPPT Temp (ºC)":dynamicdata)  [unwired: 4 in]
              n115 = Split Signals(w532) -> (→"Voltage (V)":dynamicdata, →"Voltage (V)":dynamicdata, →"Voltage (V)":dynamicdata, →"Voltage (V)":dynamicdata)  [unwired: 4 in]
              n116 = Split Signals(w530) -> (→"Current (A)":dynamicdata, →"Current (A)":dynamicdata, →"Current (A)":dynamicdata, →"Current (A)":dynamicdata)  [unwired: 4 in]
              n117 = Split Signals(w531) -> (→"Power (W)":dynamicdata, →"Power (W)":dynamicdata, →"Power (W)":dynamicdata, →"Power (W)":dynamicdata)  [unwired: 4 in]
            }
            frame #4 {
            }
          }
          n118 = local read "NET battery power (W)"() -> (w62:dbl)
          n119 = local read "Battery Charge"() -> (w61:dbl)
          "Battery Charge" <- w61
          n120 = local read "Speed (km/h)"() -> (w63:dbl)
          n121 = xnode "Formula"("BattW"=w62, "Charge%"=w61, "Speed"=w63) -> ("Result"=→"Range (km)":dbl)  [unwired: 1 in, 1 out]
        }
        n122 = local write "Status message:"("Monitoring COM port.... Press 'Disconnect' to stop listening." ("Status")) -> ()
        n123 = local read "Logfile handle"() -> (w30:refnum<file>)
        n124 = VISA Close(VISA resource name=w51, error in (no error)=w50) -> (error out=w52:errorcluster)
        n125 = Close File(refnum=w30) -> ()  [unwired: 1 in, 2 out]
        n126 = call <vilib>:"Simple Error Handler.vi"("error in (no error)"=w52) -> ()  [unwired: 4 in, 5 out]
      }
    }
    n127 = Wait (ms)(milliseconds to wait=u32 100) -> ()  [unwired: 1 out]
  }
